vi "PlaySound.vi"(8 "error in (no error)":errorcluster, 10 "Sound Type":string="startTrial", 11 "TrialBasedExperiment in":refnum<class "TrialBasedExperiment.lvclass">) -> (0 "error out":errorcluster, 3 "TrialBasedExperiment out":refnum<class "TrialBasedExperiment.lvclass">)   [LabVIEW 2010, in "TrialBasedExperiment.lvclass"]
uses:
  TrialBasedExperiment.lvclass
  Matlab API/Matlab API.lvlib
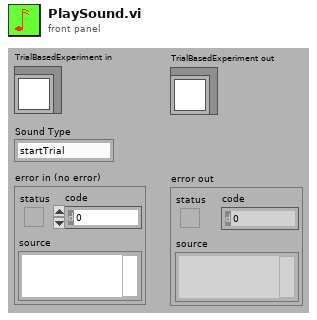
[diagram p1: front panel]
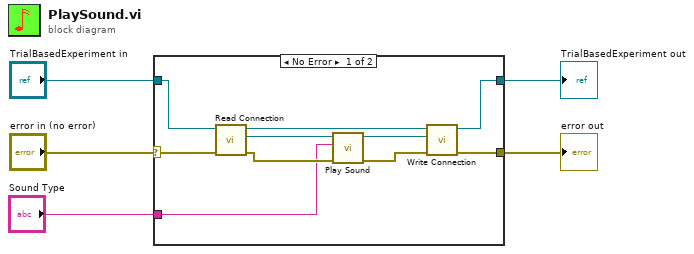
[diagram p0: block diagram]
diagram:
  n1 = case shown="No Error" "error in (no error)" {
    selector: "error in (no error)" -> [w10 w17]
    tunnel: [w8 w17] -> w4
    tunnel: [w13 w16] -> w2
    tunnel: "TrialBasedExperiment in" -> [w14 w16]
    tunnel: "Sound Type" -> [w6 _]
    frame No Error {
      n2 = call-dynamic "Read Connection.vi"("error in (no error)"=w10, "TrialBasedExperiment in"=w14) -> ("error out"=w11:errorcluster, "Connection"=w12:refnum<k5>, "TrialBasedExperiment out"=w15:refnum<class "TrialBasedExperiment.lvclass">)  [unwired: 7 in]
      n3 = call "Play Sound.vi"("error in (no error)"=w11, "Sound Type"=w6, "Matlab Connection"=w12) -> ("error out"=w9:errorcluster, "connection ID out"=w7:refnum<k5>)  [unwired: 7 out]
      n4 = call-dynamic "Write Connection.vi"("error in (no error)"=w9, "Connection"=w7, "TrialBasedExperiment in"=w15) -> ("error out"=w8:errorcluster, "TrialBasedExperiment out"=w13:refnum<class "TrialBasedExperiment.lvclass">)  [unwired: 7 in]
    }
    frame Error {
    }
  }
  "error out" <- w4
  "TrialBasedExperiment out" <- w2
